vi "Update ini Name.vi"(8 "error in (no error)":errorcluster, 10 "Plugin Name":string, 11 "configuration file path":path) -> (0 "error out":errorcluster, 3 "configuration file path Out":path)   [LabVIEW 2020]
doc: "This will rename the \"Plugin\" with Project name for Plugin name inside the ini file."
uses:
  <vilib>/Utility/config.llb/Write Key (String).vi
  <vilib>/Utility/config.llb/NI_LVConfig.lvlib
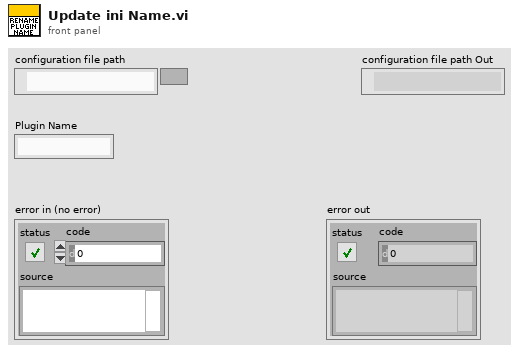
[diagram p1: front panel]
types:
  T1 = typedef "NI_LVConfig.lvlib/Config Data RefNum.ctl" = refnum<k1>
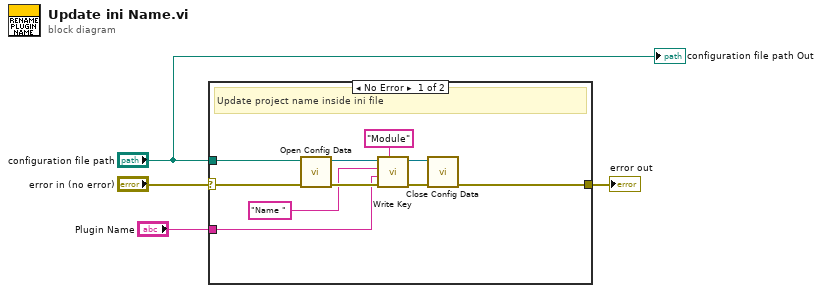
[diagram p0: block diagram]
diagram:
  n1 = case shown="No Error" "error in (no error)" {
    selector: "error in (no error)" -> [w6 w15]
    tunnel: "configuration file path" -> [w11 _]
    tunnel: "Plugin Name" -> [w7 _]
    tunnel: [w5 w15] -> w1
    frame No Error {
      # "Update project name inside ini file"
      n2 = call <vilib>:"Open Config Data.vi"("error in (no error)"=w6, "configuration file path"=w11) -> ("error out"=w10:errorcluster, "refnum"=w12:T1)  [unwired: 7 in, 1 out]
      n3 = call-poly <vilib>:"Write Key.vi"("section"="Module", "error in (no error)"=w10, "value"=w7, "key"="Name ", "refnum"=w12) -> ("error out"=w14:errorcluster, "refnum out"=w13:T1)  [unwired: 4 in, 1 out]
      n4 = call <vilib>:"Close Config Data.vi"("error in (no error)"=w14, "refnum"=w13) -> ("error out"=w5:errorcluster)  [unwired: 8 in, 1 out]
    }
    frame Error {
    }
  }
  "error out" <- w1
  "configuration file path Out" <- "configuration file path"
